vi "手动启动选择对话框.vi"() -> (2 "确定":bool, 3 "参数":T1)   [LabVIEW 2016, in "PLC.lvlib"]
uses:
  PLC.lvlib
panel:
  in  "测试模式":enum16{"正常测试", "集成干预"}(ring)
  in  "CODCr":bool
  in  "总磷总氮":bool
  in  "氨氮":bool
  in  "CODmn":bool
  in  "多参数":bool
  in  "取消":bool
  in  "确定":bool
  # "请选择启动参数"
  # "请选择启动模式："
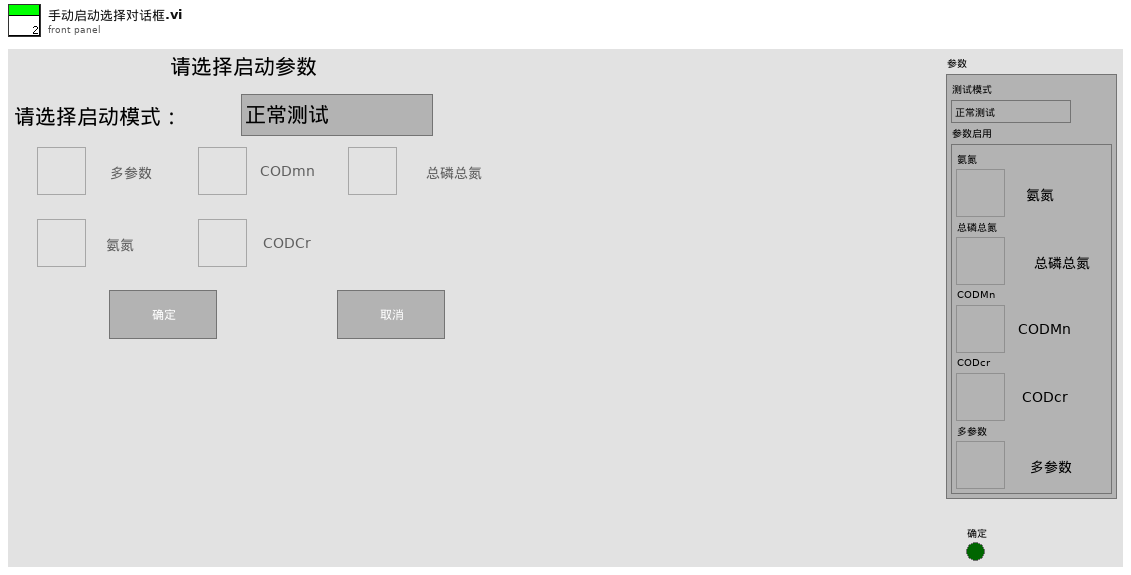
[diagram p1: front panel]
types:
  T1 = cluster{"测试模式":enum16{"正常测试", "集成干预"}, "参数启用":cluster{"氨氮":bool, "总磷总氮":bool, "CODMn":bool, "CODcr":bool, "多参数":bool}}
  T2 = enum8{"Enabled", "Disabled", "Disabled and Grayed Out"}
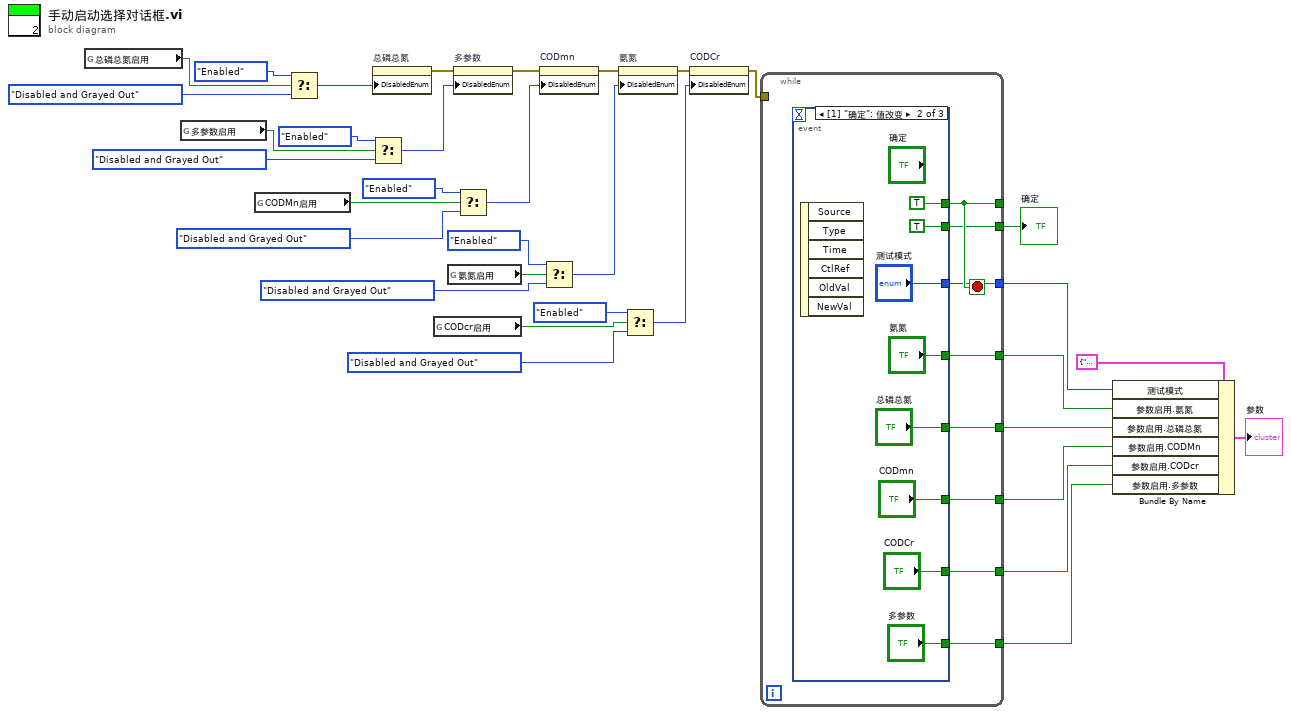
[diagram p0: block diagram]
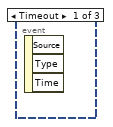
[diagram p2: hidden frame]
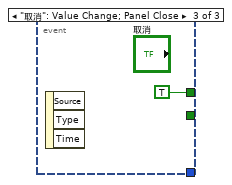
[diagram p3: hidden frame]
diagram:
  n1 = global read "系统设置全局变量.vi" "总磷总氮启用"() -> (w33:bool)
  n2 = global read "系统设置全局变量.vi" "多参数启用"() -> (w15:bool)
  n3 = global read "系统设置全局变量.vi" "CODMn启用"() -> (w19:bool)
  n4 = Select(t=T2."Enabled" ("禁用"), s=w33, f=T2."Disabled and Grayed Out" ("禁用")) -> (s? t:f=w30:T2)
  n5 = property on="总磷总氮" class="Bool (严格)"("DisabledEnum"=w30) -> (error out=w13:errorcluster)  [unwired: 2 in, 1 out]
  n6 = Select(t=T2."Enabled" ("禁用"), s=w15, f=T2."Disabled and Grayed Out" ("禁用")) -> (s? t:f=w14:T2)
  n7 = global read "系统设置全局变量.vi" "CODcr启用"() -> (w17:bool)
  n8 = global read "系统设置全局变量.vi" "氨氮启用"() -> (w21:bool)
  n9 = property on="多参数" class="Bool (严格)"(error in=w13, "DisabledEnum"=w14) -> (error out=w12:errorcluster)  [unwired: 1 in, 1 out]
  n10 = Select(t=T2."Enabled" ("禁用"), s=w19, f=T2."Disabled and Grayed Out" ("禁用")) -> (s? t:f=w18:T2)
  n11 = property on="CODmn" class="Bool (严格)"(error in=w12, "DisabledEnum"=w18) -> (error out=w11:errorcluster)  [unwired: 1 in, 1 out]
  n12 = Select(t=T2."Enabled" ("禁用"), s=w21, f=T2."Disabled and Grayed Out" ("禁用")) -> (s? t:f=w20:T2)
  n13 = property on="氨氮" class="Bool (严格)"(error in=w11, "DisabledEnum"=w20) -> (error out=w10:errorcluster)  [unwired: 1 in, 1 out]
  n14 = Select(t=T2."Enabled" ("禁用"), s=w17, f=T2."Disabled and Grayed Out" ("禁用")) -> (s? t:f=w16:T2)
  n15 = property on="CODCr" class="Bool (严格)"(error in=w10, "DisabledEnum"=w16) -> (error out=w9:errorcluster)  [unwired: 1 in, 1 out]
  n16 = while {
    tunnel: [w42] -> w1
    tunnel: [w41] -> w5
    tunnel: [w40] -> w3
    tunnel: [w39] -> _
    tunnel: [w38] -> w34
    tunnel: [w37] -> w4
    tunnel: [w36] -> w2
    tunnel: w9 -> [_]
    tunnel: [w35] -> w6
    stop <- w39 stop-if-true
    n17 = event shown="[1] \"确定\": 值改变" {
      selector: _ -> [_ _ _]
      dyn-events: _ -> [_ _ _]
      timeout: _ -> [_ _ _]
      tunnel: [_ TRUE TRUE] -> w39
      tunnel: [_ "多参数" _] -> w42
      tunnel: [_ "氨氮" _] -> w41
      tunnel: [_ "CODmn" _] -> w40
      tunnel: [_ TRUE _] -> w38
      tunnel: [_ "总磷总氮" _] -> w37
      tunnel: [_ "CODCr" _] -> w36
      tunnel: [_ "测试模式" _] -> w35
      event Timeout {
        n18 = event-data() -> ()  [unwired: 1 in, 3 out]
      }
      event "确定": Value Change {
        n19 = event-data() -> ()  [unwired: 1 in, 6 out]
      }
      event "取消": Value Change; Panel Close {
        n20 = event-data() -> ()  [unwired: 1 in, 3 out]
      }
    }
  }
  "确定" <- w34
  n21 = Bundle By Name(cluster=T1 {"测试模式"=enum."正常测试", "参数启用"={"氨氮"=FALSE, "总磷总氮"=FALSE, "CODMn"=FALSE, "CODcr"=FALSE, "多参数"=FALSE}} ("参数"), "测试模式"=w6, "参数启用.氨氮"=w5, "参数启用.总磷总氮"=w4, "参数启用.CODMn"=w3, "参数启用.CODcr"=w2, "参数启用.多参数"=w1) -> (→"参数":T1)
